vi "ma_SML Averaged Cross Spectrum.vi"(6 "reset averaging?":bool, 7 "averaging parameters":T1={"averaging type"=enum."no averaging", "averaging settings"={"weighting type"=enum."linear", "weighting settings"={"size"=10.0, "linear weighting mode"=enum."moving average"}}}, 8 "error in (no error)":errorcluster, 9 "spectral info in":T3 {"window" items=["Rectangle"=0, "Hanning"=1, "Hamming"=2, "Blackman-Harris"=3, "Exact Blackman"=4, "Blackman"=5, "Flat Top"=6, "4 Term B-Harris "=7, "7 Term B-Harris"=8, "Low Sidelobe"=9, "Blackman Nuttall"=11, "Triangle"=30, "Bartlett-Hanning"=31, "Bohman"=32, "Parzen"=33, "Welch"=34, "Kaiser"=60, "Dolph-Chebyshev"=61, "Gaussian"=62]}, 10 "FFT spectrum 2":T4 {"spectrum" format="%.2f"; "df" format="%.2f"; "f0" format="%.2f"}, 11 "FFT spectrum 1":T4 {"spectrum" format="%.2f"; "df" format="%.2f"; "f0" format="%.2f"}) -> (0 "error out":errorcluster, 1 "data ready?":bool, 2 "spectral info out":T3 {"window" items=["Rectangle"=0, "Hanning"=1, "Hamming"=2, "Blackman-Harris"=3, "Exact Blackman"=4, "Blackman"=5, "Flat Top"=6, "4 Term B-Harris "=7, "7 Term B-Harris"=8, "Low Sidelobe"=9, "Blackman Nuttall"=11, "Triangle"=30, "Bartlett-Hanning"=31, "Bohman"=32, "Parzen"=33, "Welch"=34, "Kaiser"=60, "Dolph-Chebyshev"=61, "Gaussian"=62]}, 3 "avg cross spectrum":T4 {"spectrum" format="%.2f"; "df" format="%.2f"; "f0" format="%.2f"}, 4 "averages sofar":dbl)   [LabVIEW 2020, in "NI_MAPro.lvlib"]
uses:
  NI_MAPro.lvlib
  ma_sml_Spectrum Cluster (complex).ctl
  ma_sml_Spectral Info.ctl
  ma_sml_Averaging Parameters.ctl
  ma_sml_Averaging Settings.ctl
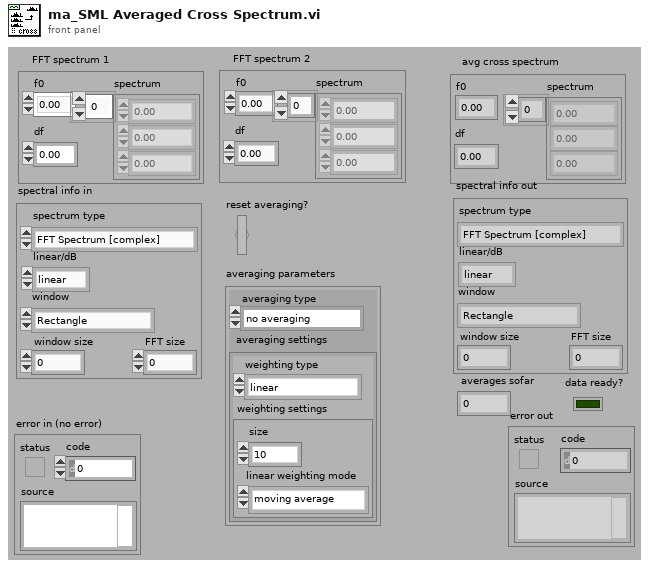
[diagram p1: front panel]
types:
  T1 = typedef "NI_MAPro.lvlib/ma_sml_Averaging Parameters.ctl" = cluster{"averaging type":enum16{"no averaging", "vector averaging", "RMS averaging", "peak hold"}, "averaging settings":T2}
  T2 = typedef "NI_MAPro.lvlib/ma_sml_Averaging Settings.ctl" = cluster{"weighting type":enum16{"linear", "exponential"}, "weighting settings":cluster{"size":dbl, "linear weighting mode":enum16{"one shot", "auto restart one shot", "moving average", "continuous"}}}
  T3 = typedef "NI_MAPro.lvlib/ma_sml_Spectral Info.ctl" = cluster{"spectrum type":enum16{"FFT Spectrum [complex]", "Amplitude [Magnitude]", "Power [Magnitude^2]", "Cross Spectrum [complex]", "Frequency Response [Complex]"}, "linear/dB":enum16{"linear", "dB"}, "window":u16, "window size":i32, "FFT size":i32}
  T4 = typedef "NI_MAPro.lvlib/ma_sml_Spectrum Cluster (complex).ctl" = cluster{"f0":dbl, "df":dbl, "spectrum":cdb[]}
  T5 = enum16{"FFT Spectrum [complex]", "Amplitude [Magnitude]", "Power [Magnitude^2]", "Cross Spectrum [complex]", "Frequency Response [Complex]"}
  T6 = enum16{"no averaging", "vector averaging", "RMS averaging", "peak hold"}
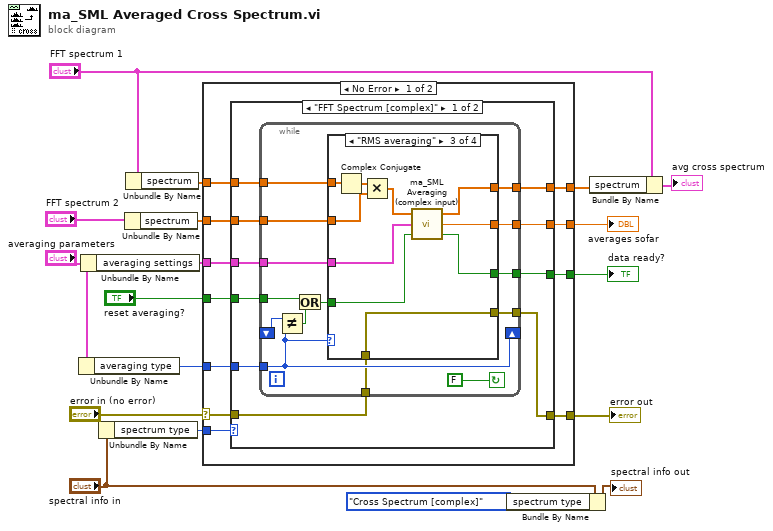
[diagram p0: block diagram]
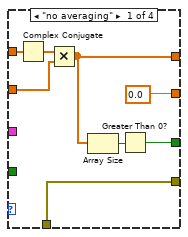
[diagram p2: hidden frame]
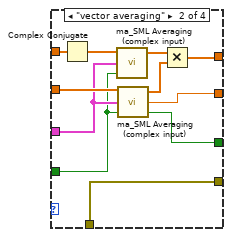
[diagram p3: hidden frame]
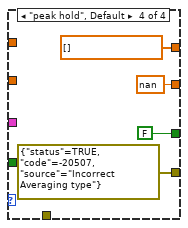
[diagram p4: hidden frame]
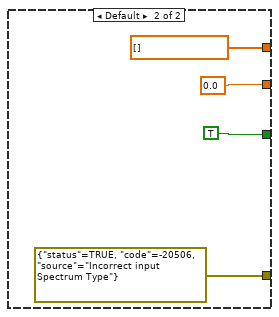
[diagram p5: hidden frame]
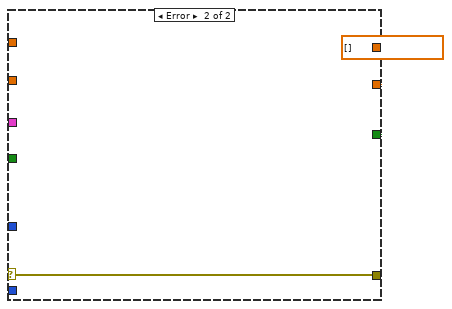
[diagram p6: hidden frame]
diagram:
  n1 = Unbundle By Name("averaging parameters") -> ("averaging type"=w4:T6)
  n2 = Unbundle By Name("averaging parameters") -> ("averaging settings"=w5:T2)
  n3 = Unbundle By Name("spectral info in") -> ("spectrum type"=w9:T5)
  n4 = Unbundle By Name("FFT spectrum 2") -> ("spectrum"=w14:cdb[])
  n5 = Unbundle By Name("FFT spectrum 1") -> ("spectrum"=w17:cdb[])
  n6 = case shown="No Error" "error in (no error)" {
    selector: "error in (no error)" -> [w19 w91]
    tunnel: [w22 FALSE] -> w15
    tunnel: [w29 0.0 ("Averaged So-far")] -> w18
    tunnel: "reset averaging?" -> [w28 _]
    tunnel: w4 -> [w27 _]
    tunnel: [w26 cdb[] [] ("Y")] -> w10
    tunnel: w17 -> [w24 _]
    tunnel: w14 -> [w23 _]
    tunnel: w5 -> [w25 _]
    tunnel: w9 -> [w21 _]
    tunnel: [w20 w91] -> w3
    frame No Error {
      n7 = case shown="\"FFT Spectrum [complex]\"" w21 {
        tunnel: [w39 0.0 ("Averaged So-far")] -> w29
        tunnel: w28 -> [w38 _]
        tunnel: w27 -> [w37 _]
        tunnel: [w36 cdb[] [] ("Y")] -> w26
        tunnel: w25 -> [w35 _]
        tunnel: w24 -> [w33 _]
        tunnel: w23 -> [w32 _]
        tunnel: [w34 TRUE] -> w22
        tunnel: [w31 errorcluster {"status"=TRUE, "code"=-20506, "source"="Incorrect input Spectrum Type"} ("error in (no error)")] -> w20
        tunnel: w19 -> [w30 _]
        frame "FFT Spectrum [complex]" {
          n8 = while {
            tunnel: w30 -> [w40]
            tunnel: [w41] -> w31
            shift-left: _ -> [w44]
            shift-right: [w43] -> _
            tunnel: w32 -> [w48]
            tunnel: w33 -> [w49]
            tunnel: [w50] -> w36
            tunnel: w37 -> [w43]
            tunnel: w38 -> [w46]
            tunnel: w35 -> [w51]
            tunnel: [w52] -> w39
            tunnel: [w53] -> w34
            stop <- FALSE continue-if-true
            n9 = Not Equal?(x=w44, y=w43) -> (x != y?=w45:bool)
            n10 = Or(x=w46, y=w45) -> (x .or. y?=w47:bool)
            n11 = case shown="\"RMS averaging\"" w43 {
              tunnel: [w55 w64 w74 FALSE ("Data Ready")] -> w53
              tunnel: [0.0 ("Averaged So-far") w65 w75 nan ("Averaged So-far")] -> w52
              tunnel: w51 -> [_ w69 w78 _]
              tunnel: w47 -> [_ w68 w77 _]
              tunnel: [w57 w63 w76 cdb[] [] ("Y")] -> w50
              tunnel: w49 -> [w59 w72 w82 _]
              tunnel: w48 -> [w58 w71 w80 _]
              tunnel: [w54 w62 w73 errorcluster {"status"=TRUE, "code"=-20507, "source"="Incorrect Averaging type"} ("error out")] -> w41
              tunnel: w40 -> [w54 w62 w73 _]
              frame "no averaging" {
                n12 = Complex Conjugate(1:w59) -> (0:w60:cdb[])
                n13 = Multiply(x=w60, y=w58) -> (x*y=w57:cdb[])
                n14 = Array Size(array=w57) -> (size(s)=w56:i32)
                n15 = Greater Than 0?(x=w56) -> (x > 0?=w55:bool)
              }
              frame "vector averaging" {
                n16 = Complex Conjugate(1:w72) -> (0:w70:cdb[])
                n17 = call "ma_SML Averaging (complex input).vi"("reset?"=w68, "averaging settings"=w69, "x"=w70) -> ("y"=w67:cdb[])  [unwired: 2 out]
                n18 = call "ma_SML Averaging (complex input).vi"("reset?"=w68, "averaging settings"=w69, "x"=w71) -> ("data ready?"=w64:bool, "averaged sofar"=w65:dbl, "y"=w66:cdb[])
                n19 = Multiply(x=w67, y=w66) -> (x*y=w63:cdb[])
              }
              frame "RMS averaging" {
                n20 = Complex Conjugate(1:w82) -> (0:w81:cdb[])
                n21 = Multiply(x=w81, y=w80) -> (x*y=w79:cdb[])
                n22 = call "ma_SML Averaging (complex input).vi"("reset?"=w77, "averaging settings"=w78, "x"=w79) -> ("data ready?"=w74:bool, "averaged sofar"=w75:dbl, "y"=w76:cdb[])
              }
              frame "peak hold", Default {
              }
            }
          }
        }
        frame Default {
        }
      }
    }
    frame Error {
    }
  }
  "averages sofar" <- w18
  "data ready?" <- w15
  "error out" <- w3
  n23 = Bundle By Name(cluster="spectral info in", "spectrum type"=T5."Cross Spectrum [complex]") -> (→"spectral info out":T3)
  n24 = Bundle By Name(cluster="FFT spectrum 1", "spectrum"=w10) -> (→"avg cross spectrum":T4)
